vi "New Stock.vi"(8 "error in (no error)":errorcluster caption="entrée d'erreur (pas d'erreur)", 10 "Parameters":T1={"Label"="", "Symbol"="SU", "Dividend"=0.0, "Currency"=enum."Euro", "ISIN"="", "Symbol_Suffix"=".PA", "Last Price"=0.0, "Dividend-Date"="", "Change (%)"=0.0}) -> (0 "error out":errorcluster caption="sortie d'erreur", 3 "Stock en sortie":refnum<class "Stock.lvclass"> caption="DNL_LabVIEW Object out")   [LabVIEW 2012, in "Stock.lvclass"]
uses:
  Stock.lvclass
  Stock Parameters.ctl
  controls/Currencies.ctl
  Stock.lvclass/Stock.ctl
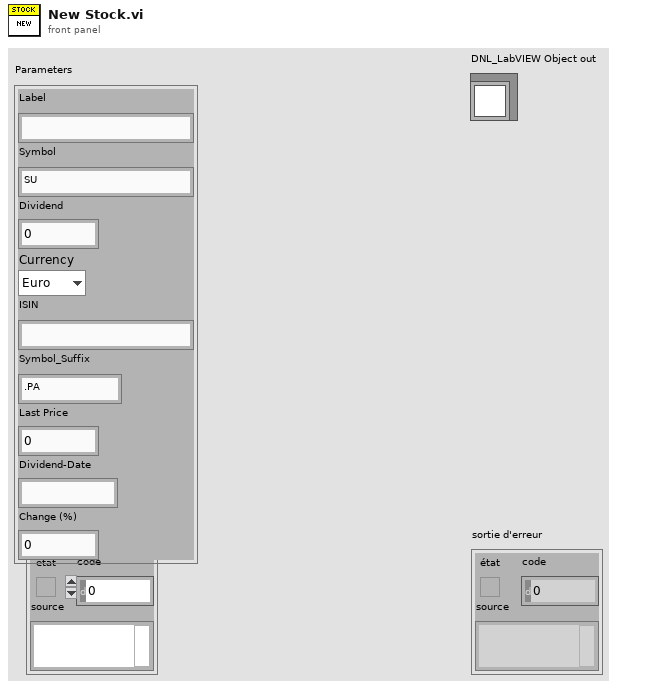
[diagram p1: front panel]
types:
  T1 = typedef "Stock.lvclass/Stock Parameters.ctl" = cluster{"Label":string, "Symbol":string, "Dividend":dbl, "Currency":T2, "ISIN":string, "Symbol_Suffix":string, "Last Price":dbl, "Dividend-Date":string, "Change (%)":dbl}
  T2 = typedef "Currencies.ctl" = enum16{"Euro", "Dollar", "Yen", "RIM", "CHF"}
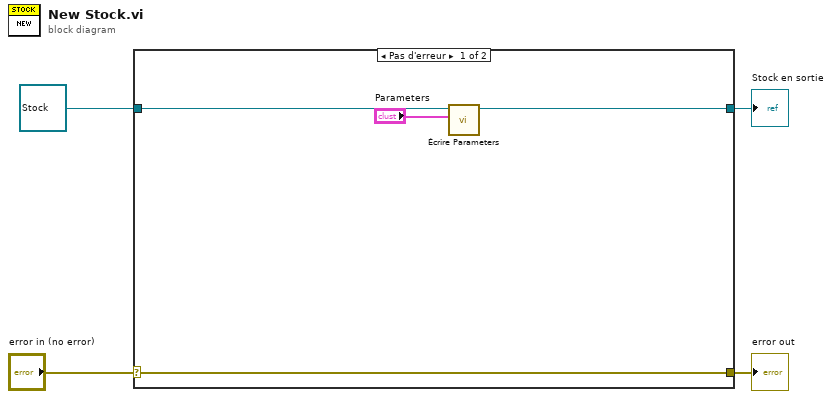
[diagram p0: block diagram]
diagram:
  n1 = case shown="Pas d'erreur" "error in (no error)" {
    selector: "error in (no error)" -> [w8 w10]
    tunnel: [w8 w10] -> w3
    tunnel: [w6 w9] -> w1
    tunnel: refnum<class "Stock.lvclass"> refnum ("Stock en entrée") -> [w7 w9]
    frame No Error {
      n2 = call "Écrire Parameters.vi"("Parameters"="Parameters", "Stock en entrée"=w7) -> ("Stock en sortie"=w6:refnum<class "Stock.lvclass">)  [unwired: 9 in]
    }
    frame Error {
    }
  }
  "error out" <- w3
  "Stock en sortie" <- w1
